vi "main_temp.vi"() -> ()   [LabVIEW 2021]
uses:
  <vilib>/Platform/TimedLoop/XDataNode/wakeup.ctl
  <vilib>/Platform/TimedLoop/XDataNode/XDNodeRunTimeDep.lvlib
  <vilib>/Platform/TimedLoop/XDataNode/nitl_modes.ctl
  <vilib>/Platform/TimedLoop/XDataNode/timing_clust.ctl
  <vilib>/Platform/TimedLoop/XDataNode/XDataNode.xnode
  <vilib>/xnet/xnet.llb/XNET Frame Type CAN.ctl
  <vilib>/xnet/xnet.llb/XNET Frame CAN.ctl
  General Purpose/references.ctl
  General Purpose/measurements.ctl
  <vilib>/xnet/xnet.llb/XNET Write (Frame CAN).vi
  <vilib>/xnet/xnet.llb/XNET Read (Frame CAN).vi
panel:
  in  "measurements":T1
  in  "references":T2
  out "CAN OUT":T3 {"payload" format="%x"; "timestamp" format="%<%.7X\n%x>T"; "type" items=["CAN Data"=0, "CAN Remote"=1, "CAN Bus Error"=2, "CAN 2.0 Data"=8, "CAN FD Data"=16, "CAN FD+BRS Data"=24, "J1939 Data"=192, "Delay"=224, "Log Trigger"=225, "Start Trigger"=226]; "identifier" format="%x"}
  in  "To ACT CH 4":bool
  in  "To ACT CH 3":bool
  in  "To ACT CH 2":bool
  out "Error 4":bool
  out "Fault 4":bool
  out "Error 3":bool
  out "Fault 3":bool
  out "Error 2":bool
  out "Fault 2":bool
  out "State code 4":i32
  out "State code 3":i32
  out "State code 2":i32
  out "State code 1":i32
  out "Error 1":bool
  out "Fault 1":bool
  in  "To ACT CH 1":bool
  in  "main stop":bool
  in  "Vdc4":dbl=750.0
  in  "Qac4":dbl
  in  "Vdc3":dbl=750.0
  in  "Qac3":dbl
  in  "Vdc2":dbl=750.0
  in  "Qac2":dbl
  in  "Emergency 4":bool
  in  "To IN OP  4":bool
  in  "SEND sp 4":bool
  in  "Clear 4":bool
  in  "Shutdwn 4":bool
  in  "Emergency 3":bool
  in  "To IN OP  3":bool
  in  "SEND sp 3":bool
  in  "Clear 3":bool
  in  "Shutdwn 3":bool
  in  "Emergency 2":bool
  in  "To IN OP  2":bool
  in  "SEND sp 2":bool
  in  "Clear 2":bool
  in  "Shutdwn 2":bool
  out "V slider 22":dbl(slide) caption="V-i" max=-10.0 scale=650.0..780.0 scale format="%#_4g"
  out "V slider 21":dbl(slide) caption="V-i" max=-10.0 scale=650.0..780.0 scale format="%#_4g"
  out "V slider 20":dbl(slide) caption="V-i" max=-10.0 scale=650.0..780.0 scale format="%#_4g"
  out "kW":dbl caption="Numeric" format="%#.3g"
  out "?VkVAr":dbl caption="Numeric" format="%.3g"
  out "kW":dbl caption="Numeric" format="%#.3g"
  out "?VkVAr":dbl caption="Numeric" format="%.3g"
  out "kW":dbl caption="Numeric" format="%#.3g"
  out "?VkVAr":dbl caption="Numeric" format="%.3g"
  out "OFF 4":bool
  out "ON 4":bool
  out "Ready 4":bool
  out "OFF 3":bool
  out "ON 3":bool
  out "Ready 3":bool
  out "OFF 2":bool
  out "ON 2":bool
  out "Ready 2":bool
  out "error out":errorcluster
  out "?VkVAr":dbl caption="Numeric" format="%.3g"
  out "kW":dbl caption="Numeric" format="%#.3g"
  out "V slider 19":dbl(slide) caption="V-i" max=-10.0 scale=650.0..780.0 scale format="%#_4g"
  in  "Vdc1":dbl=750.0
  out "OFF 1":bool
  out "ON 1":bool
  out "Ready 1":bool
  out "Numeric":i32
  out "CAN IN":T3 {"payload" format="%x"; "timestamp" format="%<%.7X\n%x>T"; "type" items=["CAN Data"=0, "CAN Remote"=1, "CAN Bus Error"=2, "CAN 2.0 Data"=8, "CAN FD Data"=16, "CAN FD+BRS Data"=24, "J1939 Data"=192, "Delay"=224, "Log Trigger"=225, "Start Trigger"=226]; "identifier" format="%x"}
  in  "newfile":bool
  in  "Log period [ms]":i64=1000
  in  "Emergency 1":bool
  in  "Qac1":dbl
  in  "conv":T5
  in  "CAN [ms]":i64=1
  out "CAN with Conv":bool
  out "Measurements":bool
  in  "Shutdwn 1":bool
  in  "Clear 1":bool
  in  "SEND sp 1":bool
  in  "To IN OP 1":bool
  out "logging":bool
  # "Resource agents: AFE 1-4"
  # "package identifiers:\n1xx VSC1 \n2xx VSC2\n3xx VSC3\n4xx VSC4\n\nx0x send from agent to resource\nx02 Power setpoints\nx06 Measurements\nx9 status\n          = [state; error; alarm; OFF; Ready; ON]\n\n \n\nx1x send from resource to agent\nx10 Power measurements\nx11 Measurements\nx12 status\n          = [state; error; alarm; full; precharge; neg; 0; 0]"
  # "B18"
  # "B22"
  # "B17"
  # "B21"
  # "B16"
  # "B20"
  # "B15"
  # "B 19\nB19"
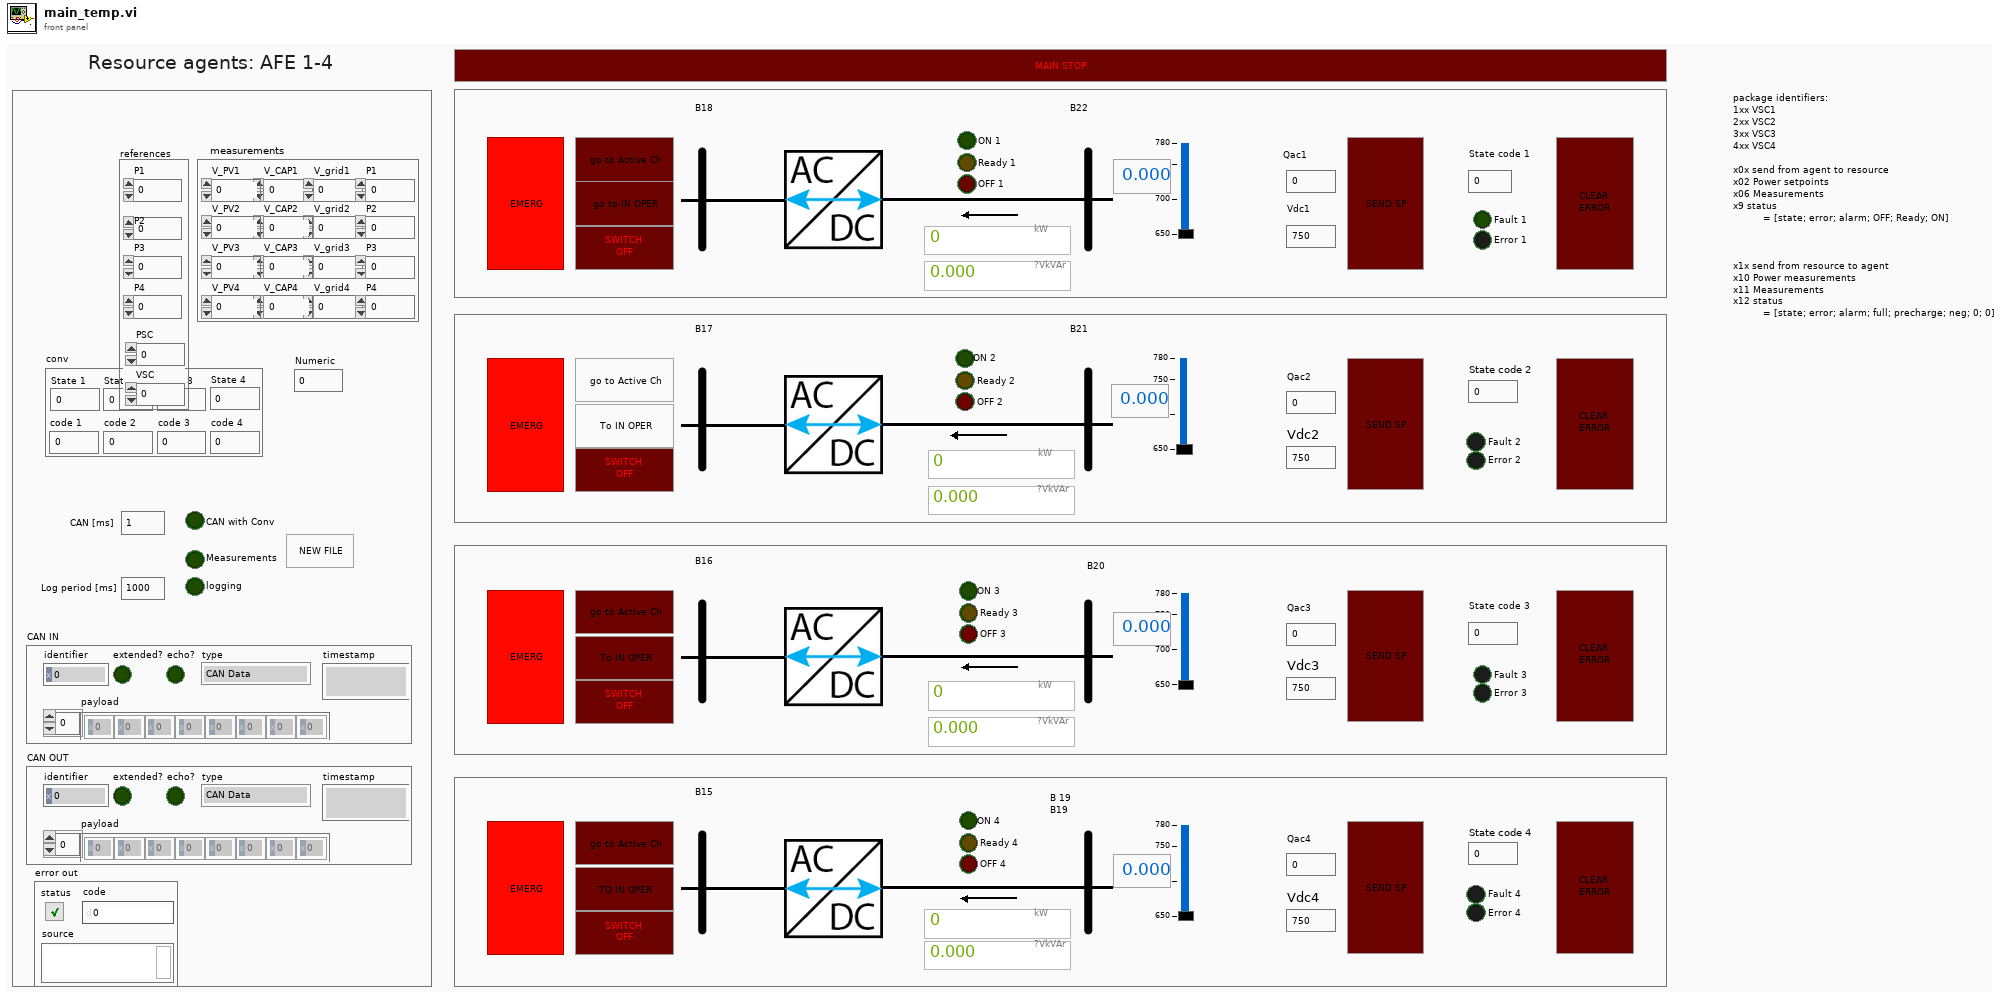
[diagram p1: front panel]
types:
  T1 = typedef "measurements.ctl" = cluster{"V_PV1":dbl, "V_CAP1":dbl, "V_PV2":dbl, "V_CAP2":dbl, "V_grid2":dbl, "V_PV3":dbl, "V_CAP3":dbl, "V_grid3":dbl, "V_PV4":dbl, "V_CAP4":dbl, "V_grid4":dbl, "V_grid1":dbl, "P1":dbl, "P2":dbl, "P3":dbl, "P4":dbl}
  T2 = typedef "references.ctl" = cluster{"P1":dbl, "\nP2":dbl, "P3":dbl, "P4":dbl, "VSC":dbl, "PSC":dbl}
  T3 = typedef "XNET Frame CAN.ctl" = cluster{"timestamp":timestamp, "payload":u8[], "identifier":u32, "type":T4, "extended?":bool, "echo?":bool}
  T4 = typedef "XNET Frame Type CAN.ctl" = u8
  T5 = cluster{"State 1":dbl, "code 1":dbl, "code 2":dbl, "code 3":dbl, "code 4":dbl, "State 2":dbl, "State 3":dbl, "State 4":dbl}
  T6 = cluster{"Frame In":refnum<k21>, "Frame Out":refnum<k21>}
  T7 = typedef "XDNodeRunTimeDep.lvlib/timing_clust.ctl" = cluster{"Expected End [f-1]":u64, "Actual End [f-1]":u64, "Finished Late? [f-1]":bool, "Expected End [i-1]":u64, "Actual End [i-1]":u64, "Finished Late? [i-1]":bool, "Expected Start [i]":u64, "Actual Start [i]":u64, "Expected Start [f]":u64, "Actual Start [f]":u64, "Source Name":string, "Structure Name":string, "Period":i64, "Deadline":i64, "Offset":i64, "Start":i64, "Priority":i32, "Timeout":i32, "Mode":T8, "Wakeup Reason":T9, "Error":errorcluster, "Source Type":string, "Secondary Source Type":string, "Global End Time":u64, "Global Start Time":u64, "Frame Duration":u64, "Iteration Duration":u64, "Assigned CPU":i32, "I/O Scan Engine Mode":u32}
  T8 = typedef "XDNodeRunTimeDep.lvlib/nitl_modes.ctl" = enum32{"No Change", "Process missed periods, maintain original phase", "Discard missed periods, maintain original phase", "Process missed periods, ignore original phase", "Discard missed periods, ignore original phase"}
  T9 = typedef "XDNodeRunTimeDep.lvlib/wakeup.ctl" = enum32{"Normal", "Aborted", "Asynchronous wakeup", "Timing source error", "Timed loop error", "Timeout"}
  T10 = cluster{"date string":string, "time string":string, "V_PV1":dbl, "P1":dbl, "Q1":dbl, "Vdc2":dbl, "P2":dbl, "Q2":dbl, "Vdc3":dbl, "P3":dbl, "Q3":dbl, "Vdc4":dbl, "P4":dbl, "Q4":dbl}
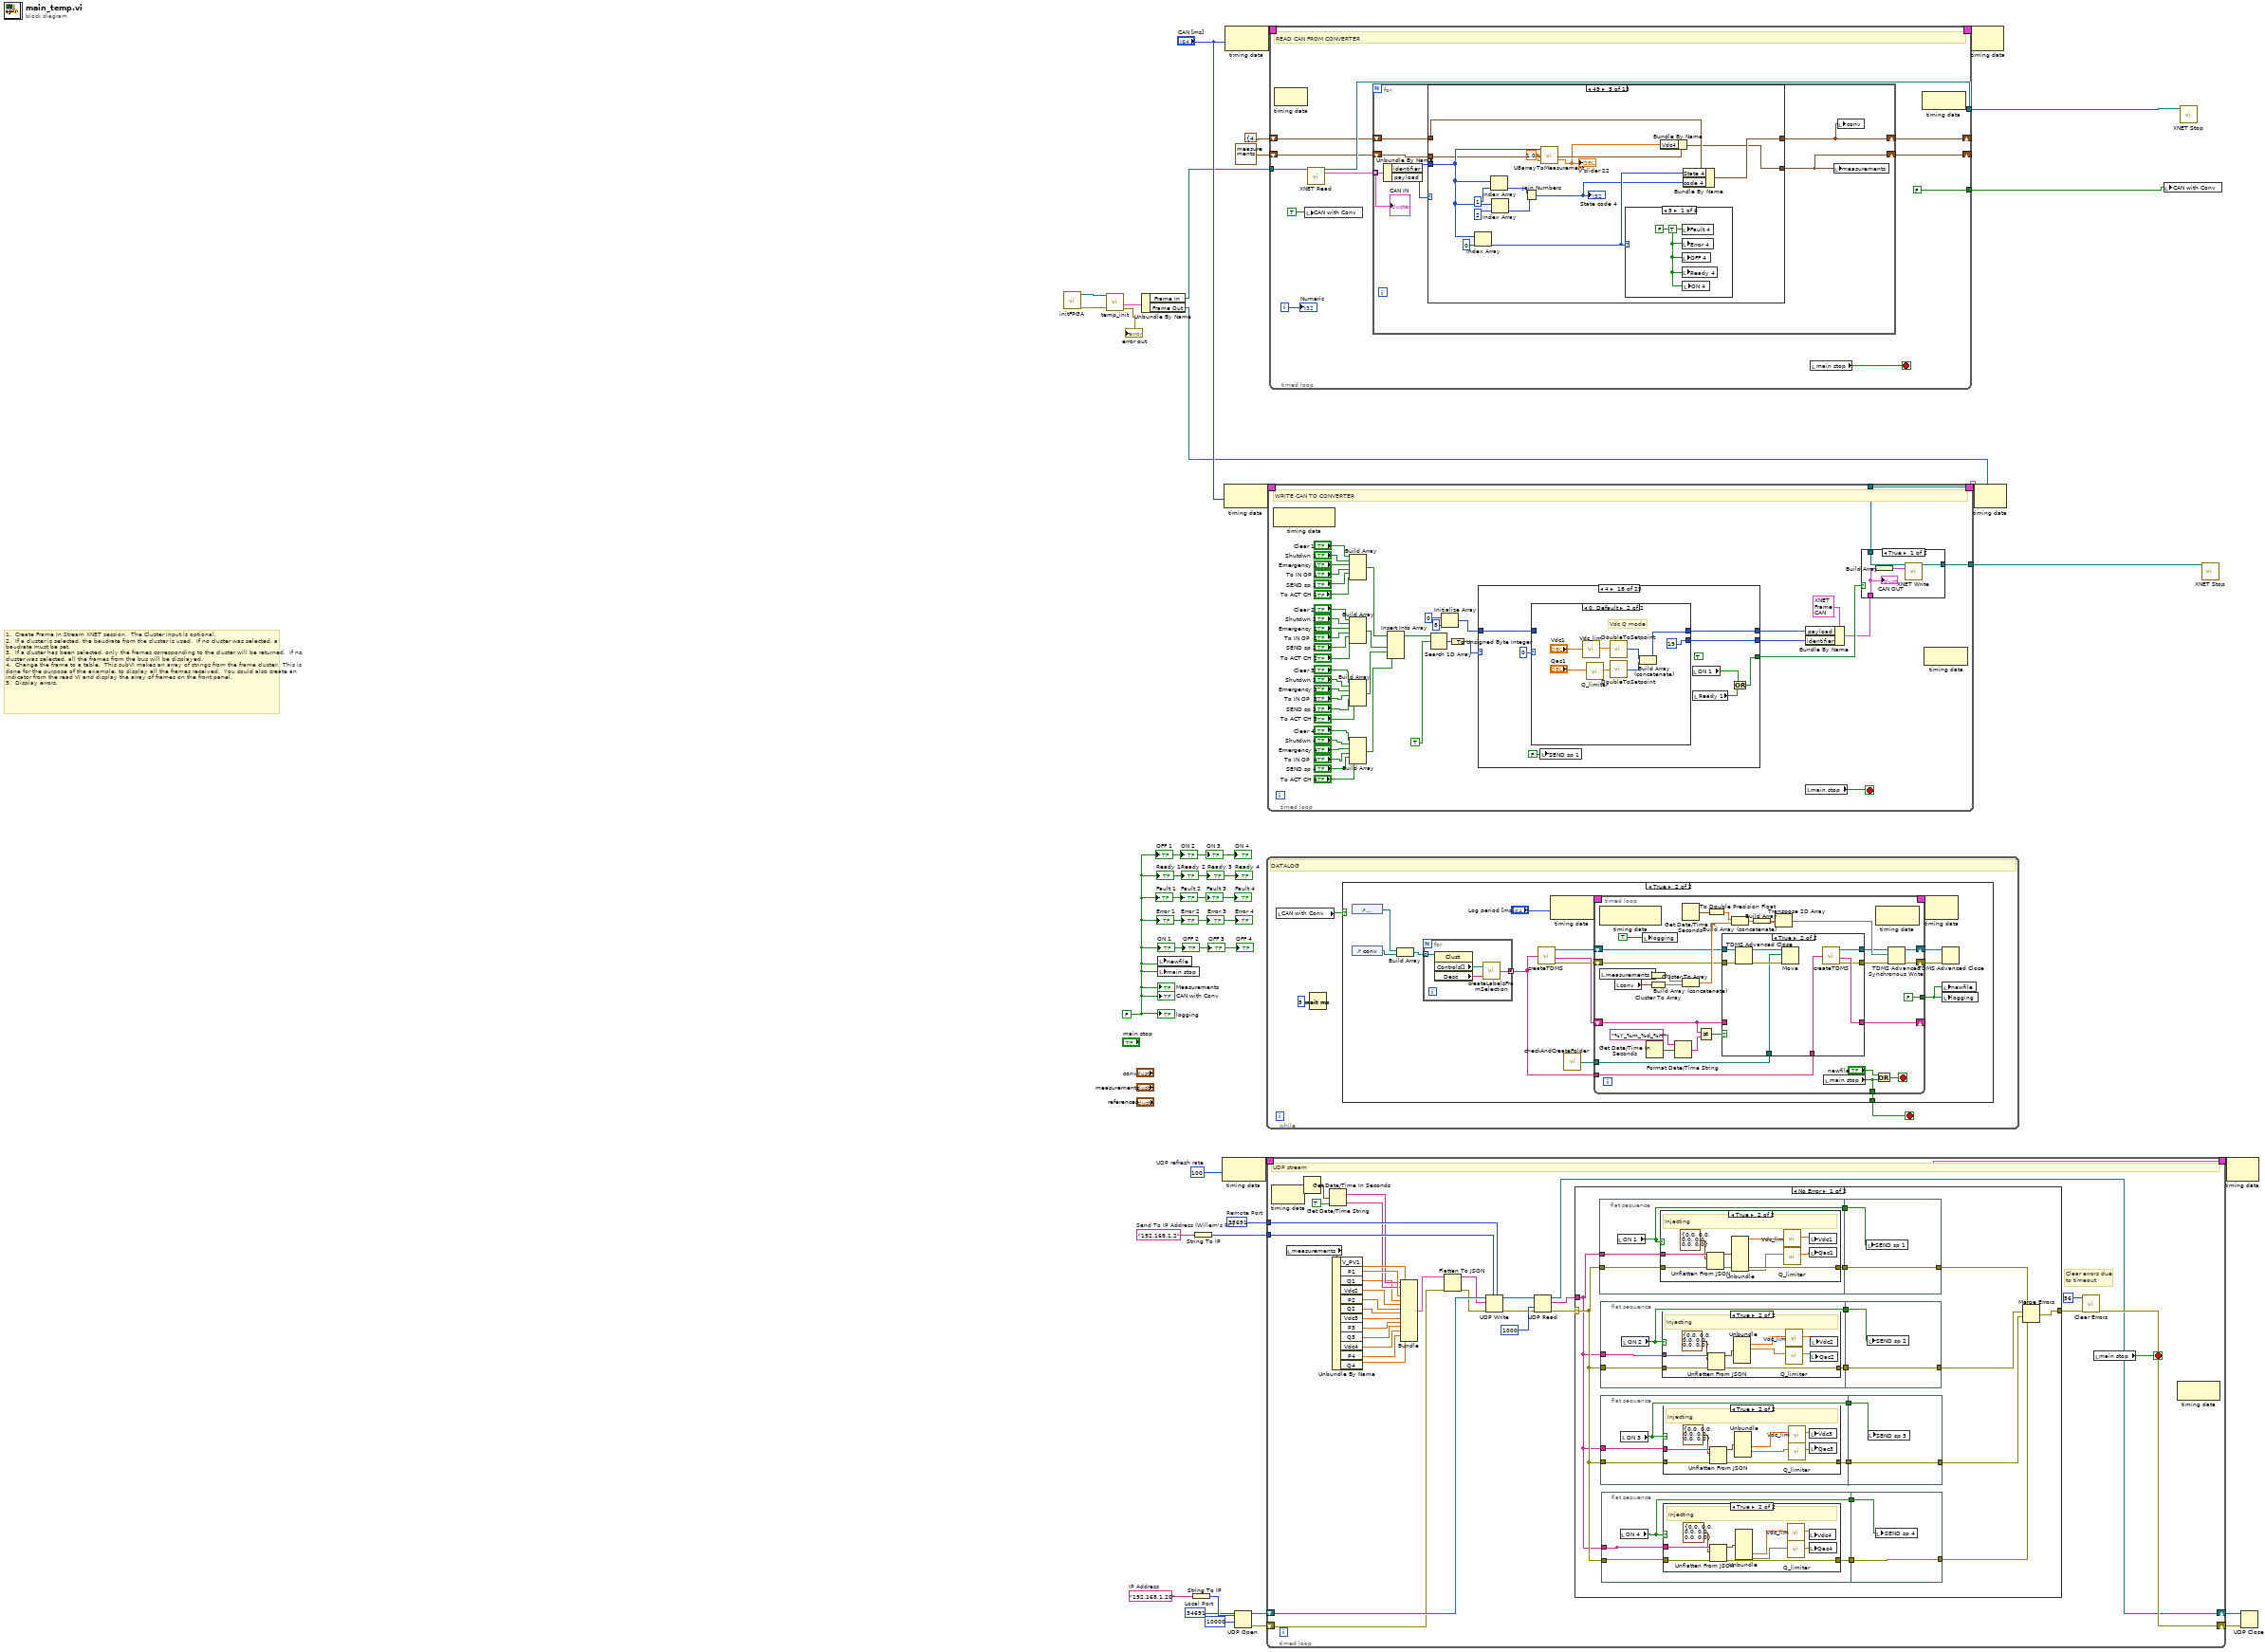
[diagram p0: block diagram]
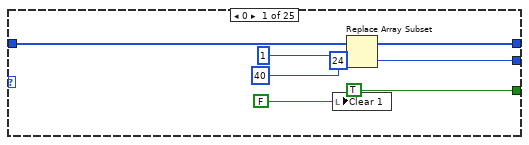
[diagram p8: hidden frame]
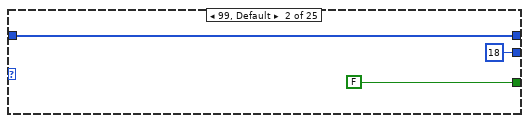
[diagram p9: hidden frame]
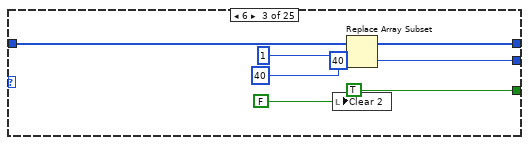
[diagram p10: hidden frame]
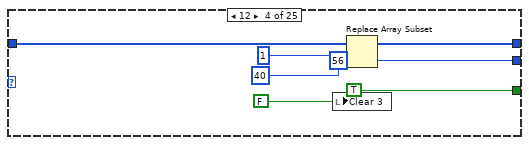
[diagram p11: hidden frame]
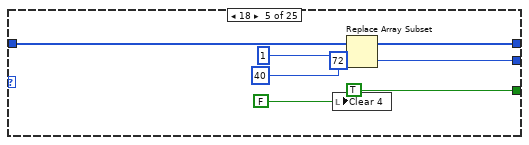
[diagram p12: hidden frame]
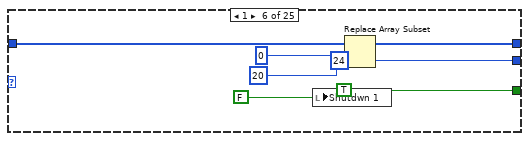
[diagram p13: hidden frame]
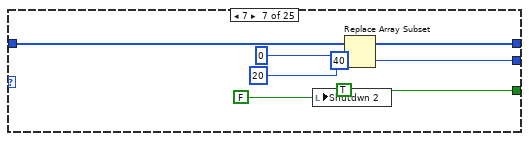
[diagram p14: hidden frame]
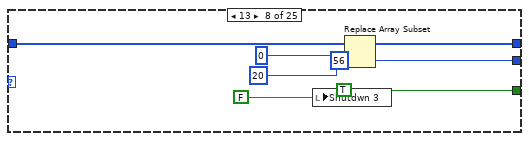
[diagram p15: hidden frame]
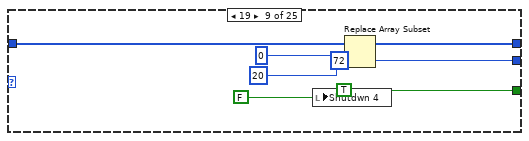
[diagram p16: hidden frame]
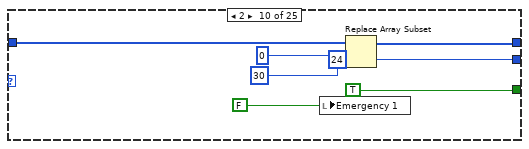
[diagram p17: hidden frame]
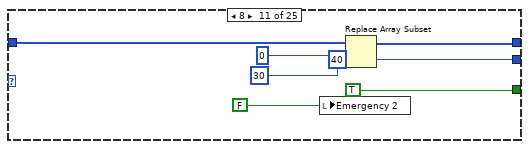
[diagram p18: hidden frame]
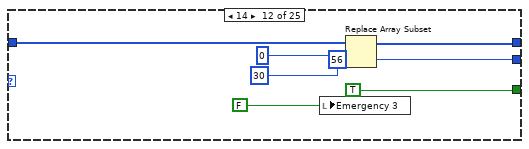
[diagram p19: hidden frame]
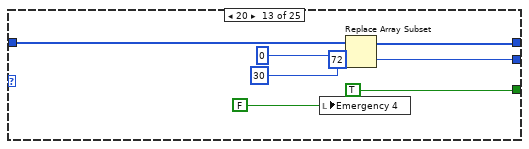
[diagram p20: hidden frame]
diagram:
  w9 = i64 100  # UDP refresh rate
  w14 = u16 34691  # Local Port
  w15 = "192.168.1.20"  # IP Address
  w5 = u16 35691  # Remote Port
  w13 = "192.168.1.2"  # Send To IP Address (Willem's PC)
  w26 = FALSE
  # "1.  Create Frame In Stream XNET session.  The Cluster input is optional.  \n2.  If a cluster is selected, the baudrate from the cluster is used.  If no cluster was selected, a baudrate must be set.\n3.  If a cluster has been selected, only the frames corresponding to the cluster will be returned.  If no cluster was selected, all the frames from the bus will be displayed.\n4.  Change the frame to a table.  This subVI makes an array of strings from the frame cluster.  This is done for the purpose of the example, to display all the frames received.  You could also create an indicator from the read VI and display the array of frames on the front panel. \n5.  Display errors."
  n1 = call "initFPGA.vi"() -> ("FPGA VI Reference Out"=w4:refnum<k20>, "error out"=w3:errorcluster)  [unwired: 4 in]
  n2 = call "temp_init.vi"("error in"=w3, "FPGA VI (in)"=w4) -> ("error out"=→"error out":errorcluster, "CAN"=w1:T6)  [unwired: 8 in]
  n3 = Unbundle By Name(w1) -> ("Frame In"=w23:refnum<k21>, "Frame Out"=w27:refnum<k21>)
  n4 = local write "newfile"(w26) -> ()
  n5 = local write "main stop"(w26) -> ()
  n6 = String To IP(1:w15) -> (0:w16:u32)
  n7 = String To IP(1:w13) -> (0:w6:u32)
  n8 = node-c288(w9) -> (w18:T7)
  n9 = node-c288("CAN [ms]") -> (w20:T7)
  n10 = node-c288("CAN [ms]") -> (w25:T7)
  n11 = UDP Open(7:w16, 9:10000 ("timeout ms (25000)"), 11:w14) -> (port=w8:refnum<k16>, 0:w7:errorcluster)  [unwired: 2 in, 1 out]
  n12 = timed-loop {
    timing: w18 -> [_]
    timing-out: [_] -> w17
    shift-right: [w49] -> w12
    shift-left: w8 -> [w65]
    shift-right: [w55] -> w11
    shift-left: w7 -> [w62]
    tunnel: w6 -> [w59]
    tunnel: w5 -> [w58]
    stop <- w57 stop-if-true
    # "Clear errors due\nto timeout"
    # "UDP stream"
    n13 = node-c288() -> ()  [unwired: 1 in, 1 out]
    n14 = local read "measurements"() -> (w44:T1)
    n15 = Get Date/Time In Seconds() -> (seconds since 1Jan1904=w48:timestamp)
    n16 = Get Date/Time String(seconds (now)=w48, want seconds? (F)=TRUE) -> (date string=w47:string, time string=w46:string)  [unwired: 1 in]
    n17 = Unbundle By Name(w44) -> ("V_PV1"=w64:dbl, "P1"=w63:dbl, "Q1"=w43:dbl, "Vdc2"=w42:dbl, "P2"=w40:dbl, "Q2"=w39:dbl, "Vdc3"=w38:dbl, "P3"=w37:dbl, "Q3"=w36:dbl, "Vdc4"=w35:dbl, "P4"=w34:dbl, "Q4"=w33:dbl)
    n18 = Bundle("date string"=w47, "time string"=w46, "V_PV1"=w64, "P1"=w63, "Q1"=w43, "Vdc2"=w42, "P2"=w40, "Q2"=w39, "Vdc3"=w38, "P3"=w37, "Q3"=w36, "Vdc4"=w35, "P4"=w34, "Q4"=w33) -> (w41:T10)  [unwired: 1 in]
    n19 = Flatten To JSON(anything=w41, error in (no error)=w62) -> (JSON string=w60:string, 11:w61:errorcluster)  [unwired: 1 in]
    n20 = UDP Write(address=w59, port or service name=w58, connection ID=w65, data in=w60, 8:w61) -> (error out=w51:errorcluster, 3:w50:refnum<k16>)  [unwired: 1 in]
    n21 = UDP Read(connection ID=w50, timeout ms (25000)=1000, 8:w51) -> (data out=w54:string, error out=w53:errorcluster, 3:w49:refnum<k16>)  [unwired: 1 in, 2 out]
    n22 = case shown="No Error" w53 {
      selector: w53 -> [w78 w145]
      tunnel: w54 -> [w77 _]
      tunnel: [w79 w145] -> w32
      frame No Error {
        n23 = flat-sequence {
          tunnel: w77 -> [w132]
          tunnel: w78 -> [w131]
          tunnel: [w130] -> w80
          tunnel: [w129] -> w66
          tunnel: w80 -> [w144]
          tunnel: [w144] -> w76
          tunnel: w66 -> [w143]
          frame #0 {
            n24 = local read "ON 1"() -> (w129:bool)
            n25 = case shown="True" w129 {
              tunnel: w132 -> [_ w142]
              tunnel: w131 -> [w133 w141]
              tunnel: [w133 w140] -> w130
              frame False {
                # "Injecting"
              }
              frame True {
                # "Injecting"
                n26 = Unflatten From JSON(JSON string=w142, type and defaults=T2 {"P1"=0.0, "\nP2"=0.0, "P3"=0.0, "P4"=0.0, "VSC"=0.0, "PSC"=0.0} ("ref"), error in (no error)=w141) -> (value=w139:T2, error out=w140:errorcluster)  [unwired: 4 in]
                n27 = Unbundle(w139) -> (w136:dbl, w134)  [unwired: 6 out]
                n28 = call "Vdc_lim.vi"("IN Vdc"=w136) -> ("OUT Vdc"=w137:dbl)  [unwired: 10 in]
                n29 = call "Q_limiter.vi"("IN Q"=w134) -> ("OUT Q"=w135:dbl)  [unwired: 10 in]
                n30 = local write "Vdc1"(w137) -> ()
                n31 = local write "Qac1"(w135) -> ()
              }
            }
          }
          frame #1 {
            n32 = local write "SEND sp 1"(w143) -> ()
          }
        }
        n33 = flat-sequence {
          tunnel: w78 -> [w116]
          tunnel: w77 -> [w114]
          tunnel: [w115] -> w70
          tunnel: [w113] -> w67
          tunnel: [w128] -> w73
          tunnel: w70 -> [w128]
          tunnel: w67 -> [w127]
          frame #0 {
            n34 = local read "ON 2"() -> (w113:bool)
            n35 = case shown="True" w113 {
              tunnel: w114 -> [_ w126]
              tunnel: w116 -> [w117 w125]
              tunnel: [w117 w124] -> w115
              frame False {
                # "Injecting"
              }
              frame True {
                # "Injecting"
                n36 = Unflatten From JSON(JSON string=w126, type and defaults=T2 {"P1"=0.0, "\nP2"=0.0, "P3"=0.0, "P4"=0.0, "VSC"=0.0, "PSC"=0.0} ("ref"), error in (no error)=w125) -> (value=w123:T2, error out=w124:errorcluster)  [unwired: 4 in]
                n37 = Unbundle(w123) -> ("P2"=w120:dbl, "P3"=w118:dbl)  [unwired: 4 out]
                n38 = call "Vdc_lim.vi"("IN Vdc"=w120) -> ("OUT Vdc"=w121:dbl)  [unwired: 10 in]
                n39 = call "Q_limiter.vi"("IN Q"=w118) -> ("OUT Q"=w119:dbl)  [unwired: 10 in]
                n40 = local write "Qac2"(w119) -> ()
                n41 = local write "Vdc2"(w121) -> ()
              }
            }
          }
          frame #1 {
            n42 = local write "SEND sp 2"(w127) -> ()
          }
        }
        n43 = flat-sequence {
          tunnel: w78 -> [w100]
          tunnel: w77 -> [w98]
          tunnel: [w99] -> w71
          tunnel: [w97] -> w68
          tunnel: [w112] -> w74
          tunnel: w71 -> [w112]
          tunnel: w68 -> [w111]
          frame #0 {
            n44 = local read "ON 3"() -> (w97:bool)
            n45 = case shown="True" w97 {
              tunnel: w98 -> [_ w110]
              tunnel: w100 -> [w101 w109]
              tunnel: [w101 w108] -> w99
              frame False {
                # "Injecting"
              }
              frame True {
                # "Injecting"
                n46 = Unflatten From JSON(JSON string=w110, type and defaults=T2 {"P1"=0.0, "\nP2"=0.0, "P3"=0.0, "P4"=0.0, "VSC"=0.0, "PSC"=0.0} ("ref"), error in (no error)=w109) -> (value=w107:T2, error out=w108:errorcluster)  [unwired: 4 in]
                n47 = Unbundle(w107) -> ("P4"=w104:dbl, "VSC"=w102:dbl)  [unwired: 4 out]
                n48 = call "Vdc_lim.vi"("IN Vdc"=w104) -> ("OUT Vdc"=w105:dbl)  [unwired: 10 in]
                n49 = call "Q_limiter.vi"("IN Q"=w102) -> ("OUT Q"=w103:dbl)  [unwired: 10 in]
                n50 = local write "Vdc3"(w105) -> ()
                n51 = local write "Qac3"(w103) -> ()
              }
            }
          }
          frame #1 {
            n52 = local write "SEND sp 3"(w111) -> ()
          }
        }
        n53 = flat-sequence {
          tunnel: w78 -> [w84]
          tunnel: [w82] -> _
          tunnel: w77 -> [w82]
          tunnel: [w83] -> w72
          tunnel: [w81] -> w69
          tunnel: [w96] -> w75
          tunnel: w72 -> [w96]
          tunnel: w69 -> [w95]
          frame #0 {
            n54 = local read "ON 4"() -> (w81:bool)
            n55 = case shown="True" w81 {
              tunnel: w82 -> [_ w94]
              tunnel: w84 -> [w85 w93]
              tunnel: [w85 w92] -> w83
              frame False {
                # "Injecting"
              }
              frame True {
                # "Injecting"
                n56 = Unflatten From JSON(JSON string=w94, type and defaults=T2 {"P1"=0.0, "\nP2"=0.0, "P3"=0.0, "P4"=0.0, "VSC"=0.0, "PSC"=0.0} ("ref"), error in (no error)=w93) -> (value=w91:T2, error out=w92:errorcluster)  [unwired: 4 in]
                n57 = Unbundle(w91) -> (w88:dbl, w87)  [unwired: 5 out]
                n58 = call "Vdc_lim.vi"("IN Vdc"=w88) -> ("OUT Vdc"=w89:dbl)  [unwired: 10 in]
                n59 = call "Q_limiter.vi"("IN Q"=w87) -> ("OUT Q"=w86:dbl)  [unwired: 10 in]
                n60 = local write "Vdc4"(w89) -> ()
                n61 = local write "Qac4"(w86) -> ()
              }
            }
          }
          frame #1 {
            n62 = local write "SEND sp 4"(w95) -> ()
          }
        }
        n63 = Merge Errors(w76, w73, w74, w75) -> (w79:errorcluster)
      }
      frame Error {
      }
    }
    n64 = call <vilib>:"Clear Errors.vi"("error in (no error)"=w32, "specific error code to clear (0: all)"=56) -> ("error out"=w55:errorcluster)  [unwired: 4 in, 1 out]
    n65 = local read "main stop"() -> (w57:bool)
    n66 = node-c288() -> ()  [unwired: 1 in, 1 out]
  }
  n67 = while {
    stop <- w150 stop-if-true
    # "DATALOG"
    n68 = local read "CAN with Conv"() -> (w148:bool)
    n69 = Wait (ms)(milliseconds to wait=u32 5) -> ()  [unwired: 1 out]
    n70 = case shown="True" w148 {
      selector: w148 -> [w151 _]
      tunnel: [w151 w164] -> w150
      frame False {
      }
      frame True {
        n71 = control-ref of="measurements"() -> (w152:refnum<vi>)
        n72 = control-ref of="conv"() -> (w157:refnum<vi>)
        n73 = Build Array(w152, w157) -> (w156:refnum<vi>[])
        n74 = for {
          tunnel: [w168] -> w155 mode=concatenating
          tunnel: w156 -> [w167] mode=indexing
          n75 = property class="Clust"(reference=w167) -> ("Controls[]"=w170:refnum<vi>[], "Desc"=w169:string)  [unwired: 1 in, 2 out]
          n76 = call "createLabelsFromSelection.vi"("log_from"=w169, "Controls[]"=w170) -> ("labels_to_log"=w168:string[])
        }
        n77 = call "createTDMS.vi"("channel name(s)"=w155) -> ("Ref"=w153:refnum<k34>, "hour"=w159:string, "error out"=w154:errorcluster)  [unwired: 3 in]
        n78 = node-c288("Log period [ms]") -> (w166:T7)
        n79 = call "checkAndCreateFolder.vi"() -> ("dup path"=w158:path)  [unwired: 1 in]
        n80 = timed-loop {
          timing: w166 -> [_]
          timing-out: [_] -> w165
          tunnel: [w190] -> w164
          tunnel: [FALSE ("logging")] -> w160
          shift-right: [w181] -> _
          shift-left: w159 -> [w180]
          tunnel: w158 -> [w179]
          tunnel: w155 -> [w178]
          shift-right: [w191] -> w161
          shift-left: w154 -> [w172]
          shift-right: [w199] -> w162
          shift-left: w153 -> [w171]
          stop <- w193 stop-if-true
          n81 = node-c288() -> ()  [unwired: 1 in, 1 out]
          n82 = local read "measurements"() -> (w177:T1)
          n83 = local read "conv"() -> (w176:T5)
          n84 = local write "logging"(TRUE ("logging")) -> ()
          n85 = Get Date/Time In Seconds() -> (seconds since 1Jan1904=w184:timestamp)
          n86 = Cluster To Array(cluster=w177) -> (array=w175:dbl[])
          n87 = Cluster To Array(cluster=w176) -> (array=w174:dbl[])
          n88 = Format Date/Time String(time format string (%c)="%Y_%m_%d_%H", seconds (now)=w184) -> (date/time string=w182:string)  [unwired: 1 in]
          n89 = Build Array (concatenate)(w175, w174) -> (w173:dbl[])
          n90 = Get Date/Time In Seconds() -> (seconds since 1Jan1904=w195:timestamp)
          n91 = Not Equal?(x=w180, y=w182) -> (x != y?=w183:bool)
          n92 = To Double Precision Float(number=w195) -> (double precision float=w194:dbl)
          n93 = case shown="True" w183 {
            tunnel: w171 -> [w202 w211]
            tunnel: [w202 w205] -> w187
            tunnel: w172 -> [w201 w210]
            tunnel: [w201 w203] -> w186
            tunnel: [w200 w204] -> w181
            tunnel: w180 -> [w200 _]
            tunnel: w179 -> [_ w207]
            tunnel: w178 -> [_ w206]
            frame False {
            }
            frame True {
              n94 = TDMS Advanced Close(8:w210, 11:w211) -> (0:w209:errorcluster, 3:w208:path)  [unwired: 2 in]
              n95 = Move(source path=w208, error in=w209, 10:w207) -> ()  [unwired: 2 in, 3 out]
              n96 = call "createTDMS.vi"("channel name(s)"=w206) -> ("Ref"=w205:refnum<k34>, "hour"=w204:string, "error out"=w203:errorcluster)  [unwired: 3 in]
            }
          }
          n97 = Build Array (concatenate)(w194, w173) -> (w198:dbl[])
          n98 = Build Array(w198) -> (w197:dbl[][])
          n99 = Transpose 2D Array(2D array=w197) -> (transposed array=w196:dbl[][])
          n100 = local read "main stop"() -> (w190:bool)
          n101 = node-c288() -> ()  [unwired: 1 in, 1 out]
          n102 = Or(x="newfile", y=w190) -> (x .or. y?=w193:bool)
          n103 = TDMS Advanced Synchronous Write(8:w186, 10:w196, 11:w187) -> (0:w191:errorcluster, 3:w199:refnum<k34>)
        }
        n104 = node-c288(w165) -> ()  [unwired: 1 out]
        n105 = TDMS Advanced Close(8:w161, 11:w162) -> ()  [unwired: 2 in, 2 out]
        n106 = local write "newfile"(w160) -> ()
        n107 = local write "logging"(w160) -> ()
      }
    }
  }
  n108 = timed-loop {
    tunnel: w27 -> [w252]
    tunnel: [w251] -> w30
    timing: w20 -> [_]
    timing-out: [_] -> w19
    stop <- w250 stop-if-true
    # "WRITE CAN TO CONVERTER"
    n109 = node-c288() -> ()  [unwired: 1 in, 1 out]
    n110 = Build Array("Clear 1", "Shutdwn 1", "Emergency 1", "To IN OP 1", "SEND sp 1", "To ACT CH 1") -> (w226:bool[])
    n111 = Build Array("Clear 2", "Shutdwn 2", "Emergency 2", "To IN OP  2", "SEND sp 2", "To ACT CH 2") -> (w225:bool[])
    n112 = Build Array("Clear 3", "Shutdwn 3", "Emergency 3", "To IN OP  3", "SEND sp 3", "To ACT CH 3") -> (w224:bool[])
    n113 = Build Array("Clear 4", "Shutdwn 4", "Emergency 4", "To IN OP  4", "SEND sp 4", "To ACT CH 4") -> (w223:bool[])
    n114 = Insert Into Array(array=w226, new element #1=w225, new element #2=w224, new element #3=w223) -> (w222:bool[])  [unwired: 1 in]
    n115 = Search 1D Array(1D array=w222, element=TRUE) -> (index of element=w244:i32)  [unwired: 1 in]
    n116 = Initialize Array(u8 0, 8 ("dimension size")) -> (w258:u8[])
    n117 = To Unsigned Byte Integer(number=w244) -> (unsigned 8bit integer=w248:u8)
    n118 = case shown="4" w248 {
      tunnel: [w272 w275 w282 w289 w296 w303 w310 w317 w324 w330 w337 w344 w351 w358 w365 w372 w379 w389 w407 w425 w443 w458 w465 w472 w479] -> w257
      tunnel: [u32 24 ("identifier") u32 18 ("identifier") u32 40 ("identifier") u32 56 ("identifier") u32 72 ("identifier") u32 24 ("identifier") u32 40 ("identifier") u32 56 ("identifier") u32 72 ("identifier") u32 24 ("identifier") u32 40 ("identifier") u32 56 ("identifier") u32 72 ("identifier") u32 24 ("identifier") u32 40 ("identifier") u32 56 ("identifier") u32 72 ("identifier") w387 w405 w423 w441 u32 24 ("identifier") u32 40 ("identifier") u32 56 ("identifier") u32 72 ("identifier")] -> w256
      tunnel: w258 -> [w270 w275 w280 w287 w294 w302 w309 w316 w323 w331 w338 w345 w352 w359 w366 w373 w380 w386 w404 w422 w440 w459 w466 w473 w480]
      tunnel: [TRUE FALSE TRUE TRUE TRUE TRUE TRUE TRUE TRUE TRUE TRUE TRUE TRUE TRUE TRUE TRUE TRUE w384 w400 w419 w436 TRUE TRUE TRUE TRUE] -> w254
      frame 0 {
        n119 = local write "Clear 1"(FALSE ("Clear")) -> ()
        n120 = Replace Array Subset(array=w270, new element=u8 40 ("new element/subarray"), index=1) -> (w272:u8[])
      }
      frame 99, Default {
      }
      frame 6 {
        n121 = local write "Clear 2"(FALSE ("Clear")) -> ()
        n122 = Replace Array Subset(array=w280, new element=u8 40 ("new element/subarray"), index=1) -> (w282:u8[])
      }
      frame 12 {
        n123 = local write "Clear 3"(FALSE ("Clear")) -> ()
        n124 = Replace Array Subset(array=w287, new element=u8 40 ("new element/subarray"), index=1) -> (w289:u8[])
      }
      frame 18 {
        n125 = local write "Clear 4"(FALSE ("Clear")) -> ()
        n126 = Replace Array Subset(array=w294, new element=u8 40 ("new element/subarray"), index=1) -> (w296:u8[])
      }
      frame 1 {
        n127 = local write "Shutdwn 1"(FALSE ("Shutdwn")) -> ()
        n128 = Replace Array Subset(array=w302, new element=u8 20 ("new element/subarray"), index=0) -> (w303:u8[])
      }
      frame 7 {
        n129 = local write "Shutdwn 2"(FALSE ("Shutdwn")) -> ()
        n130 = Replace Array Subset(array=w309, new element=u8 20 ("new element/subarray"), index=0) -> (w310:u8[])
      }
      frame 13 {
        n131 = local write "Shutdwn 3"(FALSE ("Shutdwn")) -> ()
        n132 = Replace Array Subset(array=w316, new element=u8 20 ("new element/subarray"), index=0) -> (w317:u8[])
      }
      frame 19 {
        n133 = local write "Shutdwn 4"(FALSE ("Shutdwn")) -> ()
        n134 = Replace Array Subset(array=w323, new element=u8 20 ("new element/subarray"), index=0) -> (w324:u8[])
      }
      frame 2 {
        n135 = local write "Emergency 1"(FALSE ("Idc cmd")) -> ()
        n136 = Replace Array Subset(array=w331, new element=u8 30 ("new element/subarray"), index=0) -> (w330:u8[])
      }
      frame 8 {
        n137 = local write "Emergency 2"(FALSE ("Idc cmd")) -> ()
        n138 = Replace Array Subset(array=w338, new element=u8 30 ("new element/subarray"), index=0) -> (w337:u8[])
      }
      frame 14 {
        n139 = local write "Emergency 3"(FALSE ("Idc cmd")) -> ()
        n140 = Replace Array Subset(array=w345, new element=u8 30 ("new element/subarray"), index=0) -> (w344:u8[])
      }
      frame 20 {
        n141 = local write "Emergency 4"(FALSE ("Idc cmd")) -> ()
        n142 = Replace Array Subset(array=w352, new element=u8 30 ("new element/subarray"), index=0) -> (w351:u8[])
      }
      frame 3 {
        n143 = local write "To IN OP 1"(FALSE ("Idc cmd")) -> ()
        n144 = Replace Array Subset(array=w359, new element=u8 2 ("new element/subarray"), index=0) -> (w358:u8[])
      }
      frame 9 {
        n145 = local write "To IN OP  2"(FALSE ("Idc cmd")) -> ()
        n146 = Replace Array Subset(array=w366, new element=u8 2 ("new element/subarray"), index=0) -> (w365:u8[])
      }
      frame 15 {
        n147 = local write "To IN OP  3"(FALSE ("Idc cmd")) -> ()
        n148 = Replace Array Subset(array=w373, new element=u8 2 ("new element/subarray"), index=0) -> (w372:u8[])
      }
      frame 21 {
        n149 = local write "To IN OP  4"(FALSE ("Idc cmd")) -> ()
        n150 = Replace Array Subset(array=w380, new element=u8 2 ("new element/subarray"), index=0) -> (w379:u8[])
      }
      frame 4 {
        (unwired) TRUE
        n151 = case shown="0, Default" u8 0 ("Con_State") {
          tunnel: [w390 w396] -> w389
          tunnel: [u32 16 ("identifier") u32 19 ("identifier")] -> w387
          tunnel: w386 -> [w390 _]
          frame 6 {
            # "PQ mode"
          }
          frame 0, Default {
            # "Vdc Q mode"
            n152 = call "Vdc_lim.vi"("IN Vdc"="Vdc1") -> ("OUT Vdc"=w394:dbl)  [unwired: 10 in]
            n153 = call "Q_limiter.vi"("IN Q"="Qac1") -> ("OUT Q"=w393:dbl)  [unwired: 10 in]
            n154 = call "DoubleToSetpoint.vi"("Double"=w394) -> ("SP"=w398:u8[])
            n155 = call "DoubleToSetpoint.vi"("Double"=w393) -> ("SP"=w397:u8[])
            n156 = Build Array (concatenate)(w398, w397) -> (w396:u8[])
          }
        }
        n157 = local write "SEND sp 1"(FALSE ("SEND sp")) -> ()
        n158 = local read "ON 1"() -> (w383:bool)
        n159 = local read "Ready 1"() -> (w382:bool)
        n160 = Or(x=w383, y=w382) -> (x .or. y?=w384:bool)
      }
      frame 10 {
        (unwired) TRUE
        n161 = case shown="0, Default" u8 0 ("Con_State") {
          tunnel: [w408 w414] -> w407
          tunnel: [u32 32 ("identifier") u32 35 ("identifier")] -> w405
          tunnel: w404 -> [w408 _]
          frame 6 {
            # "PQ mode"
          }
          frame 0, Default {
            # "Vdc Q mode"
            n162 = call "Vdc_lim.vi"("IN Vdc"="Vdc2") -> ("OUT Vdc"=w412:dbl)  [unwired: 10 in]
            n163 = call "Q_limiter.vi"("IN Q"="Qac2") -> ("OUT Q"=w410:dbl)  [unwired: 10 in]
            n164 = call "DoubleToSetpoint.vi"("Double"=w412) -> ("SP"=w416:u8[])
            n165 = call "DoubleToSetpoint.vi"("Double"=w410) -> ("SP"=w415:u8[])
            n166 = Build Array (concatenate)(w416, w415) -> (w414:u8[])
          }
        }
        n167 = local write "SEND sp 2"(FALSE ("SEND sp")) -> ()
        n168 = local read "ON 2"() -> (w401:bool)
        n169 = local read "Ready 2"() -> (w402:bool)
        n170 = Or(x=w401, y=w402) -> (x .or. y?=w400:bool)
      }
      frame 16 {
        (unwired) TRUE
        n171 = case shown="0, Default" u8 0 ("Con_State") {
          tunnel: [w426 w432] -> w425
          tunnel: [u32 48 ("identifier") u32 51 ("identifier")] -> w423
          tunnel: w422 -> [w426 _]
          frame 6 {
            # "PQ mode"
          }
          frame 0, Default {
            # "Vdc Q mode"
            n172 = call "Vdc_lim.vi"("IN Vdc"="Vdc3") -> ("OUT Vdc"=w431:dbl)  [unwired: 10 in]
            n173 = call "Q_limiter.vi"("IN Q"="Qac3") -> ("OUT Q"=w429:dbl)  [unwired: 10 in]
            n174 = call "DoubleToSetpoint.vi"("Double"=w431) -> ("SP"=w434:u8[])
            n175 = call "DoubleToSetpoint.vi"("Double"=w429) -> ("SP"=w433:u8[])
            n176 = Build Array (concatenate)(w434, w433) -> (w432:u8[])
          }
        }
        n177 = local write "SEND sp 3"(FALSE ("SEND sp")) -> ()
        n178 = local read "ON 3"() -> (w420:bool)
        n179 = local read "Ready 3"() -> (w418:bool)
        n180 = Or(x=w420, y=w418) -> (x .or. y?=w419:bool)
      }
      frame 22 {
        (unwired) TRUE
        n181 = case shown="0, Default" u8 0 ("Con_State") {
          tunnel: [w444 w450] -> w443
          tunnel: [u32 64 ("identifier") u32 67 ("identifier")] -> w441
          tunnel: w440 -> [w444 _]
          frame 6 {
            # "PQ mode"
          }
          frame 0, Default {
            # "Vdc Q mode"
            n182 = call "Q_limiter.vi"("IN Q"="Qac4") -> ("OUT Q"=w447:dbl)  [unwired: 10 in]
            n183 = call "Vdc_lim.vi"("IN Vdc"="Vdc4") -> ("OUT Vdc"=w448:dbl)  [unwired: 10 in]
            n184 = call "DoubleToSetpoint.vi"("Double"=w448) -> ("SP"=w452:u8[])
            n185 = call "DoubleToSetpoint.vi"("Double"=w447) -> ("SP"=w451:u8[])
            n186 = Build Array (concatenate)(w452, w451) -> (w450:u8[])
          }
        }
        n187 = local write "SEND sp 4"(FALSE ("SEND sp")) -> ()
        n188 = local read "ON 4"() -> (w437:bool)
        n189 = local read "Ready 4"() -> (w438:bool)
        n190 = Or(x=w437, y=w438) -> (x .or. y?=w436:bool)
      }
      frame 5 {
        n191 = local write "To ACT CH 1"(FALSE ("Idc cmd")) -> ()
        n192 = Replace Array Subset(array=w459, new element=u8 1 ("new element/subarray"), index=0) -> (w458:u8[])
      }
      frame 11 {
        n193 = local write "To ACT CH 2"(FALSE ("Idc cmd")) -> ()
        n194 = Replace Array Subset(array=w466, new element=u8 1 ("new element/subarray"), index=0) -> (w465:u8[])
      }
      frame 17 {
        n195 = local write "To ACT CH 3"(FALSE ("Idc cmd")) -> ()
        n196 = Replace Array Subset(array=w473, new element=u8 1 ("new element/subarray"), index=0) -> (w472:u8[])
      }
      frame 23 {
        n197 = local write "To ACT CH 4"(FALSE ("Idc cmd")) -> ()
        n198 = Replace Array Subset(array=w480, new element=u8 1 ("new element/subarray"), index=0) -> (w479:u8[])
      }
    }
    n199 = Bundle By Name(cluster=T3 {"timestamp"=timestamp(0 s since 1904-01-01), "payload"=[], "identifier"=0, "type"=0, "extended?"=FALSE, "echo?"=FALSE} ("CAN frame 3"), "payload"=w257, "identifier"=w256) -> (w253:T3)
    n200 = local read "main stop"() -> (w250:bool)
    n201 = case shown="True" w254 {
      tunnel: w253 -> [w266 _]
      tunnel: w252 -> [w264 _]
      tunnel: [w263 _] -> w251
      frame True {
        n202 = Build Array(w266) -> (w265:T3[])
        n203 = call-poly <vilib>:"XNET Write.vi"("session in"=w264, "data"=w265) -> ("session out"=w263:refnum<k21>)  [unwired: 12 in, 1 out]
        "CAN OUT" <- w266
      }
      frame False {
      }
    }
    n204 = node-c288() -> ()  [unwired: 1 in, 1 out]
  }
  n205 = timed-loop {
    timing: w25 -> [_]
    timing-out: [_] -> w24
    tunnel: w23 -> [w484]
    tunnel: [w491] -> w31
    shift-right: [w486] -> _
    shift-left: T5 {"State 1"=4.0, "code 1"=0.0, "code 2"=0.0, "code 3"=0.0, "code 4"=0.0, "State 2"=4.0, "State 3"=4.0, "State 4"=4.0} ("Conv 2") -> [w490]
    tunnel: [FALSE ("stop CAN")] -> w28
    shift-right: [w482] -> _
    shift-left: T1 {"V_PV1"=0.0, "V_CAP1"=0.0, "V_PV2"=0.0, "V_CAP2"=0.0, "V_grid2"=0.0, "V_PV3"=0.0, "V_CAP3"=0.0, "V_grid3"=0.0, "V_PV4"=0.0, "V_CAP4"=0.0, "V_grid4"=0.0, "V_grid1"=0.0, "P1"=0.0, "P2"=0.0, "P3"=0.0, "P4"=0.0} ("measurements 2") -> [w483]
    i -> [w485]
    stop <- w489 stop-if-true
    # "READ CAN FROM CONVERTER"
    n206 = node-c288() -> ()  [unwired: 1 in, 1 out]
    n207 = local write "CAN with Conv"(TRUE) -> ()
    n208 = call-poly <vilib>:"XNET Read.vi"("session in"=w484) -> ("session out"=w491:refnum<k21>, "data"=w492:T3[])  [unwired: 11 in, 2 out]
    n209 = for {
      tunnel: w492 -> [w497] mode=indexing
      shift-right: [w495] -> w486
      shift-left: w490 -> [w496]
      shift-right: [w493] -> w482
      shift-left: w483 -> [w494]
      n210 = Unbundle By Name(w497) -> ("identifier"=w499:u32, "payload"=w498:u8[])
      n211 = case shown="49" w499 {
        tunnel: w498 -> [_ w506 w531 w556 w581 w607 w613 w619 w625 w630 w638 w646 w654]
        tunnel: w496 -> [w501 w514 w539 w564 w589 w605 w611 w617 w623 w628 w634 w643 w651]
        tunnel: [w501 w513 w538 w563 w588 w605 w611 w617 w623 w628 w634 w643 w651] -> w495
        tunnel: w494 -> [w500 w503 w528 w553 w579 w602 w608 w614 w620 w626 w633 w642 w649]
        tunnel: [w500 w504 w529 w554 w580 w602 w608 w614 w620 w627 w632 w641 w650] -> w493
        frame 0, Default {
        }
        frame 25 {
          w502 = 1.0 ("factor 1")
          n212 = Index Array(array=w506, index=0) -> (element=w507:u8)
          n213 = call "U8arrayToMeasurement.vi"("factor 2"=w502, "factor 1"=w502, "payload"=w506) -> ("Meas 2"=w505:dbl)  [unwired: 1 out]
          "V slider 19" <- w505
          n214 = Index Array(array=w506, index=1) -> (element=w510:u8)
          n215 = Index Array(array=w506, index=2) -> (element=w509:u8)
          n216 = Join Numbers(hi=w510, lo=w509) -> ((hi.lo)=w508:u16)
          "State code 1" <- w508
          n217 = Bundle By Name(cluster=w503, "V_PV1"=w505) -> (w504:T1)
          n218 = case shown="5" w507 {
            frame 5 {
              w517 = FALSE ("Fault 1")
              n219 = local write "Fault 1"(TRUE ("Fault 1")) -> ()
              n220 = local write "Error 1"(w517) -> ()
              n221 = local write "OFF 1"(w517) -> ()
              n222 = local write "Ready 1"(w517) -> ()
              n223 = local write "ON 1"(w517) -> ()
            }
            frame 1 {
              w518 = FALSE ("Fault 1")
              n224 = local write "Fault 1"(w518) -> ()
              n225 = local write "Error 1"(TRUE ("Error 1")) -> ()
              n226 = local write "OFF 1"(w518) -> ()
              n227 = local write "Ready 1"(w518) -> ()
              n228 = local write "ON 1"(w518) -> ()
            }
            frame 2 {
              w521 = FALSE ("Fault 1")
              n229 = local write "Fault 1"(w521) -> ()
              n230 = local write "Error 1"(w521) -> ()
              n231 = local write "OFF 1"(TRUE ("OFF 1")) -> ()
              n232 = local write "Ready 1"(w521) -> ()
              n233 = local write "ON 1"(w521) -> ()
            }
            frame 3 {
              w523 = FALSE ("Fault 1")
              n234 = local write "Fault 1"(w523) -> ()
              n235 = local write "Error 1"(w523) -> ()
              n236 = local write "OFF 1"(w523) -> ()
              n237 = local write "Ready 1"(TRUE ("Ready 1")) -> ()
              n238 = local write "ON 1"(w523) -> ()
            }
            frame 4 {
              w525 = FALSE ("Fault 1")
              n239 = local write "Fault 1"(w525) -> ()
              n240 = local write "Error 1"(w525) -> ()
              n241 = local write "OFF 1"(w525) -> ()
              n242 = local write "Ready 1"(w525) -> ()
              n243 = local write "ON 1"(TRUE ("ON 1")) -> ()
            }
            frame 99, Default {
              w526 = FALSE ("Fault 1")
              n244 = local write "Fault 1"(w526) -> ()
              n245 = local write "Error 1"(w526) -> ()
              n246 = local write "OFF 1"(w526) -> ()
              n247 = local write "Ready 1"(w526) -> ()
              n248 = local write "ON 1"(w526) -> ()
            }
          }
          n249 = Bundle By Name(cluster=w514, "State 1"=w507, "code 1"=w508) -> (w513:T5)
        }
        frame 41 {
          w527 = 1.0 ("factor 1")
          n250 = call "U8arrayToMeasurement.vi"("factor 2"=w527, "factor 1"=w527, "payload"=w531) -> ("Meas 2"=w530:dbl)  [unwired: 1 out]
          "V slider 20" <- w530
          n251 = Index Array(array=w531, index=0) -> (element=w537:u8)
          n252 = Index Array(array=w531, index=1) -> (element=w534:u8)
          n253 = Index Array(array=w531, index=2) -> (element=w533:u8)
          n254 = Join Numbers(hi=w534, lo=w533) -> ((hi.lo)=w532:u16)
          "State code 2" <- w532
          n255 = Bundle By Name(cluster=w528, "Vdc2"=w530) -> (w529:T1)
          n256 = case shown="5" w537 {
            frame 5 {
              w542 = FALSE ("Fault 1")
              n257 = local write "Fault 2"(TRUE ("Fault 1")) -> ()
              n258 = local write "Error 2"(w542) -> ()
              n259 = local write "OFF 2"(w542) -> ()
              n260 = local write "Ready 2"(w542) -> ()
              n261 = local write "ON 2"(w542) -> ()
            }
            frame 1 {
              w543 = FALSE ("Fault 1")
              n262 = local write "Fault 2"(w543) -> ()
              n263 = local write "Error 2"(TRUE ("Error 1")) -> ()
              n264 = local write "OFF 2"(w543) -> ()
              n265 = local write "Ready 2"(w543) -> ()
              n266 = local write "ON 2"(w543) -> ()
            }
            frame 2 {
              w546 = FALSE ("Fault 1")
              n267 = local write "Fault 2"(w546) -> ()
              n268 = local write "Error 2"(w546) -> ()
              n269 = local write "OFF 2"(TRUE ("OFF 1")) -> ()
              n270 = local write "Ready 2"(w546) -> ()
              n271 = local write "ON 2"(w546) -> ()
            }
            frame 3 {
              w548 = FALSE ("Fault 1")
              n272 = local write "Fault 2"(w548) -> ()
              n273 = local write "Error 2"(w548) -> ()
              n274 = local write "OFF 2"(w548) -> ()
              n275 = local write "Ready 2"(TRUE ("Ready 1")) -> ()
              n276 = local write "ON 2"(w548) -> ()
            }
            frame 4 {
              w550 = FALSE ("Fault 1")
              n277 = local write "Fault 2"(w550) -> ()
              n278 = local write "Error 2"(w550) -> ()
              n279 = local write "OFF 2"(w550) -> ()
              n280 = local write "Ready 2"(w550) -> ()
              n281 = local write "ON 2"(TRUE ("ON 1")) -> ()
            }
            frame 99, Default {
              w551 = FALSE ("Fault 1")
              n282 = local write "Fault 2"(w551) -> ()
              n283 = local write "Error 2"(w551) -> ()
              n284 = local write "OFF 2"(w551) -> ()
              n285 = local write "Ready 2"(w551) -> ()
              n286 = local write "ON 2"(w551) -> ()
            }
          }
          n287 = Bundle By Name(cluster=w539, "State 2"=w537, "code 2"=w532) -> (w538:T5)
        }
        frame 57 {
          w552 = 1.0 ("factor 1")
          n288 = Index Array(array=w556, index=0) -> (element=w562:u8)
          n289 = Index Array(array=w556, index=1) -> (element=w559:u8)
          n290 = Index Array(array=w556, index=2) -> (element=w558:u8)
          n291 = call "U8arrayToMeasurement.vi"("factor 2"=w552, "factor 1"=w552, "payload"=w556) -> ("Meas 2"=w555:dbl)  [unwired: 1 out]
          "V slider 21" <- w555
          n292 = Join Numbers(hi=w559, lo=w558) -> ((hi.lo)=w557:u16)
          "State code 3" <- w557
          n293 = case shown="5" w562 {
            frame 5 {
              w567 = FALSE ("Fault 1")
              n294 = local write "Fault 3"(TRUE ("Fault 1")) -> ()
              n295 = local write "Error 3"(w567) -> ()
              n296 = local write "OFF 3"(w567) -> ()
              n297 = local write "Ready 3"(w567) -> ()
              n298 = local write "ON 3"(w567) -> ()
            }
            frame 1 {
              w568 = FALSE ("Fault 1")
              n299 = local write "Fault 3"(w568) -> ()
              n300 = local write "Error 3"(TRUE ("Error 1")) -> ()
              n301 = local write "OFF 3"(w568) -> ()
              n302 = local write "Ready 3"(w568) -> ()
              n303 = local write "ON 3"(w568) -> ()
            }
            frame 2 {
              w571 = FALSE ("Fault 1")
              n304 = local write "Fault 3"(w571) -> ()
              n305 = local write "Error 3"(w571) -> ()
              n306 = local write "OFF 3"(TRUE ("OFF 1")) -> ()
              n307 = local write "Ready 3"(w571) -> ()
              n308 = local write "ON 3"(w571) -> ()
            }
            frame 3 {
              w573 = FALSE ("Fault 1")
              n309 = local write "Fault 3"(w573) -> ()
              n310 = local write "Error 3"(w573) -> ()
              n311 = local write "OFF 3"(w573) -> ()
              n312 = local write "Ready 3"(TRUE ("Ready 1")) -> ()
              n313 = local write "ON 3"(w573) -> ()
            }
            frame 4 {
              w575 = FALSE ("Fault 1")
              n314 = local write "Fault 3"(w575) -> ()
              n315 = local write "Error 3"(w575) -> ()
              n316 = local write "OFF 3"(w575) -> ()
              n317 = local write "Ready 3"(w575) -> ()
              n318 = local write "ON 3"(TRUE ("ON 1")) -> ()
            }
            frame 99, Default {
              w576 = FALSE ("Fault 1")
              n319 = local write "Fault 3"(w576) -> ()
              n320 = local write "Error 3"(w576) -> ()
              n321 = local write "OFF 3"(w576) -> ()
              n322 = local write "Ready 3"(w576) -> ()
              n323 = local write "ON 3"(w576) -> ()
            }
          }
          n324 = Bundle By Name(cluster=w553, "Vdc3"=w555) -> (w554:T1)
          n325 = Bundle By Name(cluster=w564, "State 3"=w562, "code 3"=w557) -> (w563:T5)
        }
        frame 73 {
          w577 = 1.0 ("factor 1")
          n326 = Index Array(array=w581, index=0) -> (element=w587:u8)
          n327 = Index Array(array=w581, index=1) -> (element=w584:u8)
          n328 = Index Array(array=w581, index=2) -> (element=w583:u8)
          n329 = Join Numbers(hi=w584, lo=w583) -> ((hi.lo)=w582:u16)
          "State code 4" <- w582
          n330 = call "U8arrayToMeasurement.vi"("factor 2"=w577, "factor 1"=w577, "payload"=w581) -> ("Meas 2"=w578:dbl)  [unwired: 1 out]
          "V slider 22" <- w578
          n331 = case shown="5" w587 {
            frame 5 {
              w592 = FALSE ("Fault 1")
              n332 = local write "Fault 4"(TRUE ("Fault 1")) -> ()
              n333 = local write "Error 4"(w592) -> ()
              n334 = local write "OFF 4"(w592) -> ()
              n335 = local write "Ready 4"(w592) -> ()
              n336 = local write "ON 4"(w592) -> ()
            }
            frame 1 {
              w593 = FALSE ("Fault 1")
              n337 = local write "Fault 4"(w593) -> ()
              n338 = local write "Error 4"(TRUE ("Error 1")) -> ()
              n339 = local write "OFF 4"(w593) -> ()
              n340 = local write "Ready 4"(w593) -> ()
              n341 = local write "ON 4"(w593) -> ()
            }
            frame 2 {
              w596 = FALSE ("Fault 1")
              n342 = local write "Fault 4"(w596) -> ()
              n343 = local write "Error 4"(w596) -> ()
              n344 = local write "OFF 4"(TRUE ("OFF 1")) -> ()
              n345 = local write "Ready 4"(w596) -> ()
              n346 = local write "ON 4"(w596) -> ()
            }
            frame 3 {
              w598 = FALSE ("Fault 1")
              n347 = local write "Fault 4"(w598) -> ()
              n348 = local write "Error 4"(w598) -> ()
              n349 = local write "OFF 4"(w598) -> ()
              n350 = local write "Ready 4"(TRUE ("Ready 1")) -> ()
              n351 = local write "ON 4"(w598) -> ()
            }
            frame 4 {
              w600 = FALSE ("Fault 1")
              n352 = local write "Fault 4"(w600) -> ()
              n353 = local write "Error 4"(w600) -> ()
              n354 = local write "OFF 4"(w600) -> ()
              n355 = local write "Ready 4"(w600) -> ()
              n356 = local write "ON 4"(TRUE ("ON 1")) -> ()
            }
            frame 99, Default {
              w601 = FALSE ("Fault 1")
              n357 = local write "Fault 4"(w601) -> ()
              n358 = local write "Error 4"(w601) -> ()
              n359 = local write "OFF 4"(w601) -> ()
              n360 = local write "Ready 4"(w601) -> ()
              n361 = local write "ON 4"(w601) -> ()
            }
          }
          n362 = Bundle By Name(cluster=w579, "Vdc4"=w578) -> (w580:T1)
          n363 = Bundle By Name(cluster=w589, "State 4"=w587, "code 4"=w582) -> (w588:T5)
        }
        frame 258 {
          w606 = 1000.0 ("factor 1")
          # "Q"
          # "P"
          n364 = call "U8arrayToMeasurement.vi"("factor 2"=w606, "factor 1"=w606, "payload"=w607) -> ("Meas 2"=→"?VkVAr":dbl, "Meas 1"=→"kW":dbl)
        }
        frame 514 {
          w612 = 1000.0 ("factor 1")
          # "Q"
          # "P"
          n365 = call "U8arrayToMeasurement.vi"("factor 2"=w612, "factor 1"=w612, "payload"=w613) -> ("Meas 2"=→"?VkVAr":dbl, "Meas 1"=→"kW":dbl)
        }
        frame 770 {
          w618 = 1000.0 ("factor 1")
          # "Q"
          # "P"
          n366 = call "U8arrayToMeasurement.vi"("factor 2"=w618, "factor 1"=w618, "payload"=w619) -> ("Meas 2"=→"?VkVAr":dbl, "Meas 1"=→"kW":dbl)
        }
        frame 1026 {
          w624 = 1000.0 ("factor 1")
          # "Q"
          # "P"
          n367 = call "U8arrayToMeasurement.vi"("factor 2"=w624, "factor 1"=w624, "payload"=w625) -> ("Meas 2"=→"?VkVAr":dbl, "Meas 1"=→"kW":dbl)
        }
        frame 262 {
          w631 = 1.0 ("factor 1")
          n368 = call "U8arrayToMeasurement.vi"("factor 2"=w631, "factor 1"=w631, "payload"=w630) -> ("Meas 1"=w629:dbl)  [unwired: 1 out]
          n369 = Bundle By Name(cluster=w626, "V_PV1"=w629) -> (w627:T1)
        }
        frame 518 {
          w639 = 1.0 ("factor 1")
          # "Vdc"
          n370 = call "U8arrayToMeasurement.vi"("factor 2"=w639, "factor 1"=w639, "payload"=w638) -> ("Meas 2"=w636:dbl, "Meas 1"=w637:dbl)
          n371 = Add(x=w637, y=w636) -> (x+y=w635:dbl)
          n372 = Bundle By Name(cluster=w633, "Vdc2"=w635) -> (w632:T1)
        }
        frame 774 {
          w647 = 1.0 ("factor 1")
          # "Vdc"
          n373 = call "U8arrayToMeasurement.vi"("factor 2"=w647, "factor 1"=w647, "payload"=w646) -> ("Meas 2"=w644:dbl, "Meas 1"=w645:dbl)
          n374 = Add(x=w645, y=w644) -> (x+y=w640:dbl)
          n375 = Bundle By Name(cluster=w642, "Vdc3"=w640) -> (w641:T1)
        }
        frame 1030 {
          w655 = 1.0 ("factor 1")
          # "Vdc"
          n376 = call "U8arrayToMeasurement.vi"("factor 2"=w655, "factor 1"=w655, "payload"=w654) -> ("Meas 2"=w652:dbl, "Meas 1"=w653:dbl)
          n377 = Add(x=w653, y=w652) -> (x+y=w648:dbl)
          n378 = Bundle By Name(cluster=w649, "Vdc4"=w648) -> (w650:T1)
        }
      }
      n379 = local write "measurements"(w493) -> ()
      n380 = local write "conv"(w495) -> ()
      "CAN IN" <- w497
    }
    n381 = local read "main stop"() -> (w489:bool)
    n382 = node-c288() -> ()  [unwired: 1 in, 1 out]
    "Numeric" <- w485
  }
  n383 = node-c288(w24) -> ()  [unwired: 1 out]
  n384 = node-c288(w19) -> ()  [unwired: 1 out]
  n385 = local write "CAN with Conv"(w28) -> ()
  n386 = call <vilib>:"XNET Stop.vi"("session in"=w31) -> ()  [unwired: 13 in, 2 out]
  n387 = call <vilib>:"XNET Stop.vi"("session in"=w30) -> ()  [unwired: 13 in, 2 out]
  n388 = node-c288(w17) -> ()  [unwired: 1 out]
  n389 = UDP Close(connection ID=w12, 8:w11) -> ()  [unwired: 2 out]
  "Measurements" <- w26
  "CAN with Conv" <- w26
  "logging" <- w26
  "Ready 1" <- w26
  "ON 1" <- w26
  "OFF 1" <- w26
  "Ready 2" <- w26
  "ON 2" <- w26
  "OFF 2" <- w26
  "Ready 4" <- w26
  "ON 4" <- w26
  "OFF 4" <- w26
  "ON 3" <- w26
  "Ready 3" <- w26
  "OFF 3" <- w26
  "Fault 1" <- w26
  "Error 1" <- w26
  "Fault 2" <- w26
  "Error 2" <- w26
  "Fault 3" <- w26
  "Error 3" <- w26
  "Fault 4" <- w26
  "Error 4" <- w26
